vi "Newmark-ReadArguments.vi"(0 "Table VRN IN":refnum<visa-resource-name>, 1 "N_Args":i32, 11 "Error IN":errorcluster, 12 "Timeout (ms)":u32) -> (3 "N_Found":i32, 4 "Table VRN OUT":refnum<visa-resource-name>, 6 "Args":string[](array[string]), 10 "Error":bool, 14 "Exception":string, 15 "Error OUT":errorcluster)   [LabVIEW 2019]
panel:
  out "Fermeture":bool
  out "Ouverture":bool
  out "Exception":i32
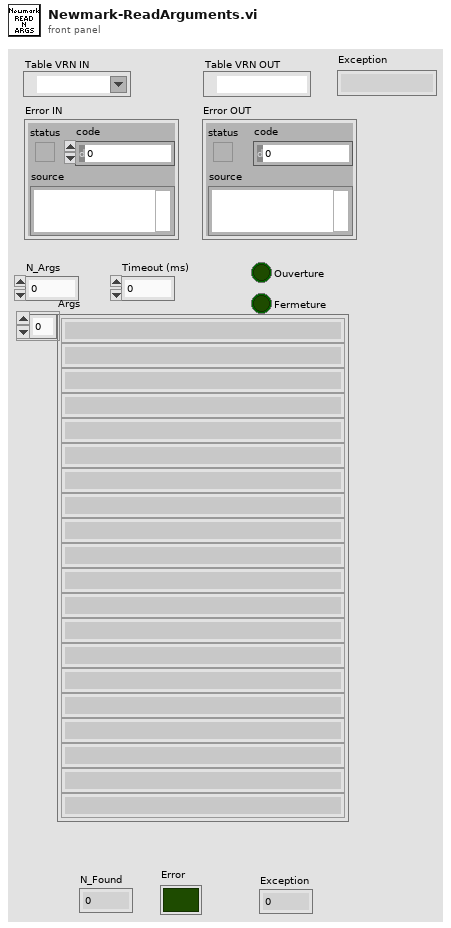
[diagram p1: front panel]
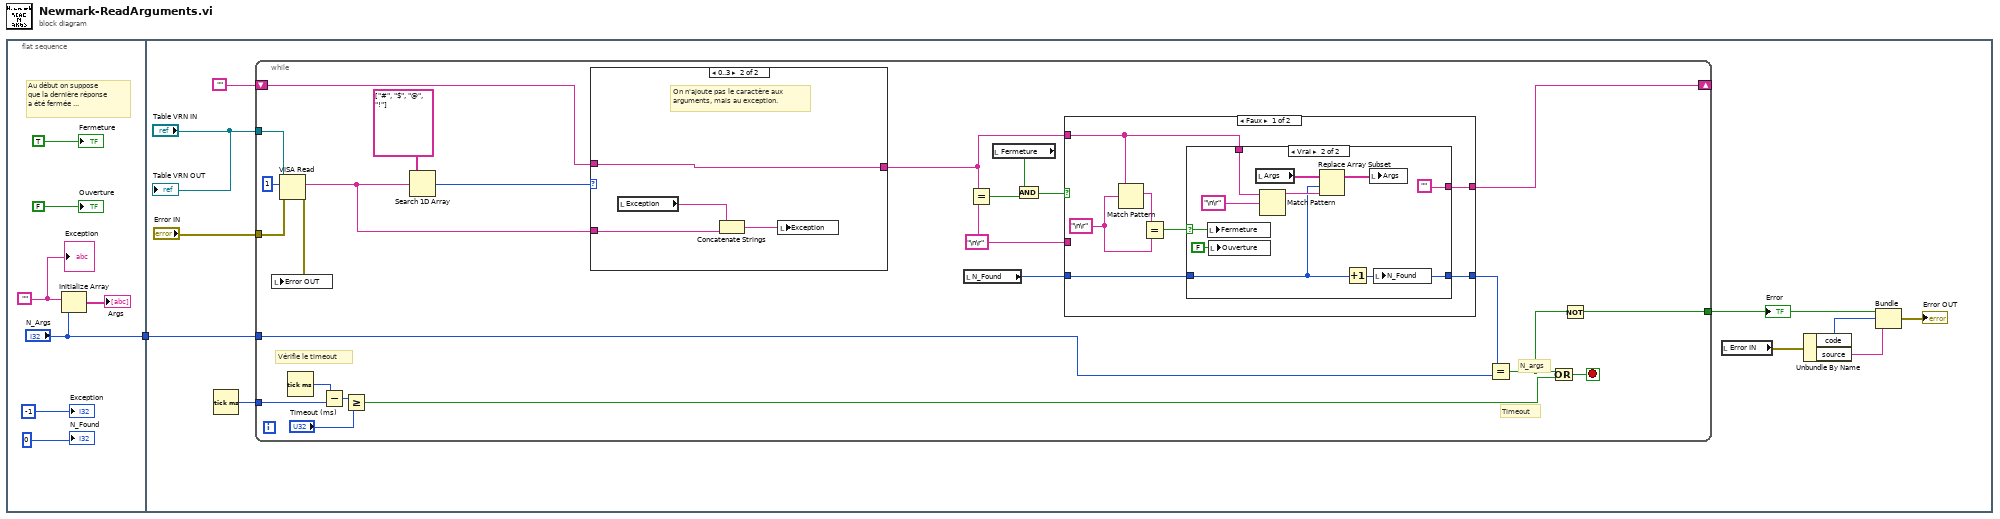
[diagram p0: block diagram]
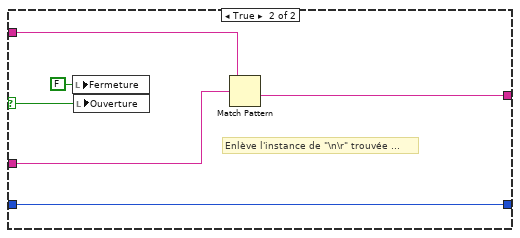
[diagram p3: hidden frame]
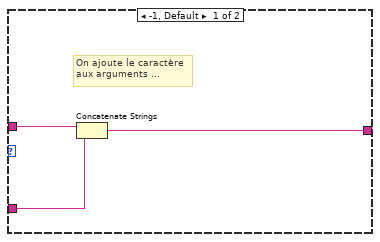
[diagram p4: hidden frame]
diagram:
  n1 = flat-sequence {
    tunnel: ["N_Args"] -> w1
    tunnel: w1 -> [w15]
    frame #0 {
      w2 = ""
      # "Au début on suppose\nque la dernière réponse\na été fermée ..."
      n2 = Initialize Array(w2, "N_Args") -> (→"Args":string[])
      "Fermeture" <- TRUE
      "Ouverture" <- FALSE ("Ouverture")
      "N_Found" <- 0 ("N_Found")
      "Exception" <- -1 ("Exception")
      "Exception" <- w2
    }
    frame #1 {
      n3 = Tick Count (ms)() -> (millisecond timer value=w17:u32)
      n4 = while {
        tunnel: "Table VRN IN" -> [w43]
        tunnel: "Error IN" -> [w42]
        tunnel: w17 -> [w39]
        tunnel: w15 -> [w36]
        shift-right: [w26] -> _
        shift-left: "" -> [w34]
        tunnel: [w23] -> w13
        stop <- w35 stop-if-true
        w25 = "\n\r"
        # "N_args"
        # "Timeout"
        # "Vérifie le timeout"
        n5 = VISA Read(VISA resource name=w43, byte count=u32 1, error in (no error)=w42) -> (read buffer=w20:string, error out=w22:errorcluster)  [unwired: 2 out]
        n6 = local write "Error OUT"(w22) -> ()
        n7 = Tick Count (ms)() -> (millisecond timer value=w40:u32)
        n8 = Subtract(x=w40, y=w39) -> (x-y=w38:u32)
        n9 = Greater Or Equal?(x=w38, y="Timeout (ms)") -> (x >= y?=w24:bool)
        n10 = Search 1D Array(1D array=string[] ["#", "$", "@", "!"], element=w20) -> (index of element=w19:i32)  [unwired: 1 in]
        n11 = case shown="0..3" w19 {
          tunnel: w20 -> [w70 w74]
          tunnel: w34 -> [w71 w75]
          tunnel: [w69 w75] -> w30
          frame -1, Default {
            # "On ajoute le caractère\naux arguments ..."
            n12 = Concatenate Strings(w71, w70) -> (w69:string)
          }
          frame 0..3 {
            # "On n'ajoute pas le caractère aux\narguments, mais au exception."
            n13 = local read "Exception"() -> (w73:string)
            n14 = Concatenate Strings(w73, w74) -> (w72:string)
            n15 = local write "Exception"(w72) -> ()
          }
        }
        n16 = local read "N_Found"() -> (w28:i32)
        n17 = Equal?(x=w30, y=w25) -> (x = y?=w33:bool)
        n18 = local read "Fermeture"() -> (w32:bool)
        n19 = And(x=w32, y=w33) -> (x .and. y?=w31:bool)
        n20 = case shown="Faux" w31 {
          selector: w31 -> [_ w68]
          tunnel: w30 -> [w47 w65]
          tunnel: [w46 w63] -> w26
          tunnel: [w45 w66] -> w29
          tunnel: w28 -> [w44 w66]
          tunnel: w25 -> [_ w64]
          frame False {
            w49 = "\n\r"
            n21 = Match Pattern(string=w47, regular expression=w49) -> (match substring=w50:string)  [unwired: 1 in, 3 out]
            n22 = Equal?(x=w50, y=w49) -> (x = y?=w48:bool)
            n23 = case shown="Vrai" w48 {
              selector: w48 -> [_ w62]
              tunnel: w47 -> [w52 w59]
              tunnel: [w52 ""] -> w46
              tunnel: [w51 w60] -> w45
              tunnel: w44 -> [w51 w53]
              frame False {
              }
              frame True {
                n24 = local write "Fermeture"(w62) -> ()
                n25 = local write "Ouverture"(FALSE ("Ouverture")) -> ()
                n26 = local read "Args"() -> (w56:string[])
                n27 = Match Pattern(string=w59, regular expression="\n\r") -> (before substring=w55:string)  [unwired: 1 in, 3 out]
                n28 = Replace Array Subset(array=w56, new element=w55, index=w53) -> (w54:string[])
                n29 = Increment(x=w53) -> (x+1=w60:i32)
                n30 = local write "Args"(w54) -> ()
                n31 = local write "N_Found"(w60) -> ()
              }
            }
          }
          frame True {
            # "Enlève l'instance de \"\\n\\r\" trouvée ..."
            n32 = local write "Fermeture"(FALSE ("Fermeture")) -> ()
            n33 = local write "Ouverture"(w68) -> ()
            n34 = Match Pattern(string=w65, regular expression=w64) -> (after substring=w63:string)  [unwired: 1 in, 3 out]
          }
        }
        n35 = Equal?(x=w29, y=w36) -> (x = y?=w27:bool)
        n36 = Or(x=w27, y=w24) -> (x .or. y?=w35:bool)
        n37 = Not(x=w27) -> (.not. x?=w23:bool)
      }
      "Error" <- w13
      n38 = local read "Error IN"() -> (w14:errorcluster)
      n39 = Unbundle By Name(w14) -> ("code"=w12:i32, "source"=w11:string)
      n40 = Bundle(w13, "code"=w12, "source"=w11) -> (→"Error OUT":cluster{bool, "code":i32, "source":string})  [unwired: 1 in]
      "Table VRN OUT" <- "Table VRN IN"
    }
  }
